vi "generate_write.vi"(10 "to Write":u64 format="%x", 11 "Command":T1=enum."Read FIFO") -> (2 "data to write":u64 format="%x", 3 "data to write string":string)   [LabVIEW 2020]
uses:
  VNA-Commands.ctl
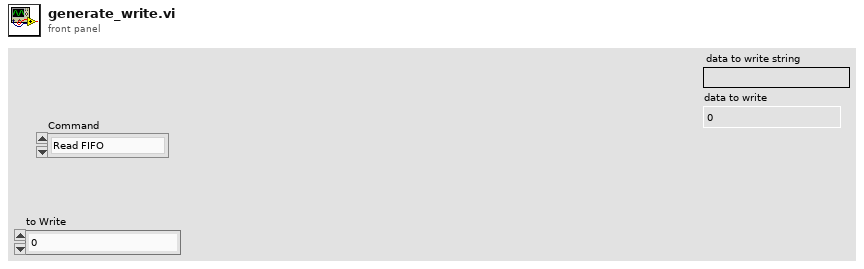
[diagram p1: front panel]
types:
  T1 = typedef "VNA-Commands.ctl" = enum16{"Nop", "Indicate", "Read 1B", "Read 2B", "Read 4B", "Read 8B", "Read FIFO", "Write 1B", "Write 2B", "Write 4B", "Write 8B", "Write FIFO"}
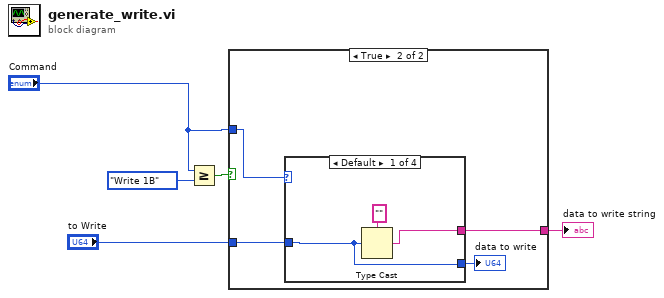
[diagram p0: block diagram]
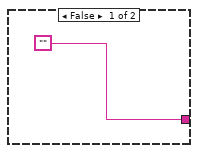
[diagram p2: hidden frame]
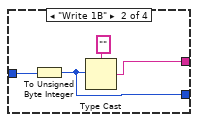
[diagram p3: hidden frame]
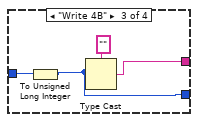
[diagram p4: hidden frame]
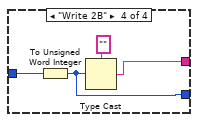
[diagram p5: hidden frame]
diagram:
  n1 = Greater Or Equal?(x="Command", y=VNA-Commands."Write 1B") -> (x >= y?=w4:bool)
  n2 = case shown="True" w4 {
    tunnel: ["" w8] -> w3
    tunnel: "to Write" -> [_ w9]
    tunnel: "Command" -> [_ w10]
    frame False {
    }
    frame True {
      n3 = case shown="Default" w10 {
        tunnel: w9 -> [w11 w15 w19 w23]
        tunnel: [w12 w16 w20 w24] -> w8
        tunnel: [w11 w14 w18 w22] -> w7
        frame Default {
          n4 = Type Cast(type="", x=w11) -> (*(type *) &x=w12:string)
        }
        frame "Write 1B" {
          n5 = To Unsigned Byte Integer(number=w15) -> (unsigned 8bit integer=w14:u8)
          n6 = Type Cast(type="", x=w14) -> (*(type *) &x=w16:string)
        }
        frame "Write 4B" {
          n7 = To Unsigned Long Integer(number=w19) -> (unsigned 32bit integer=w18:u32)
          n8 = Type Cast(type="", x=w18) -> (*(type *) &x=w20:string)
        }
        frame "Write 2B" {
          n9 = To Unsigned Word Integer(number=w23) -> (unsigned 16bit integer=w22:u16)
          n10 = Type Cast(type="", x=w22) -> (*(type *) &x=w24:string)
        }
      }
      "data to write" <- w7
    }
  }
  "data to write string" <- w3
